vi "Register .NET Events.vi"(8 "error in":errorcluster, 11 "MyEventGrid in":refnum<class "MyEventGrid.lvclass">) -> (0 "error out":errorcluster, 3 "MyEventGrid out":refnum<class "MyEventGrid.lvclass">)   [LabVIEW 2024]
uses:
  MyEventGrid.lvclass
  source/Grid/SourceGrid.lvclass/SourceGrid.ctl
  MyEventGrid.lvclass/MyEventGrid.ctl
  D:/git/Sourcegrid-LabVIEW/source/Grid/SourceGrid.lvclass
  D:/git/Sourcegrid-LabVIEW/tests/MyEventGrid/MyEventGrid.lvclass
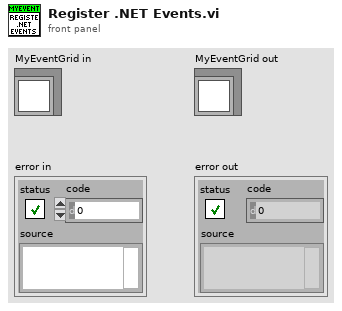
[diagram p1: front panel]
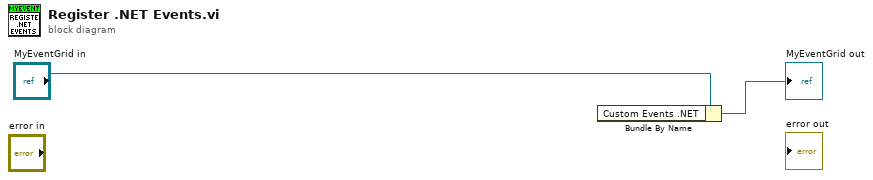
[diagram p0: block diagram]
diagram:
  n1 = Bundle By Name(cluster="MyEventGrid in") -> (→"MyEventGrid out":refnum<class "MyEventGrid.lvclass">, "Custom Events .NET"=w4:refnum<k27>)
